vi "Funnel_ToolPath_Testing.vi"() -> ()   [LabVIEW 2020]
panel:
  out "XY Graph 2":cluster{cluster{dbl, dbl}[]}[](graph)
  out "Array":cluster{dbl, dbl}[](array[cluster])
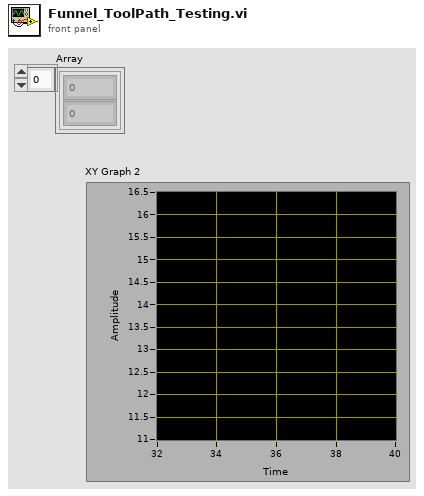
[diagram p1: front panel]
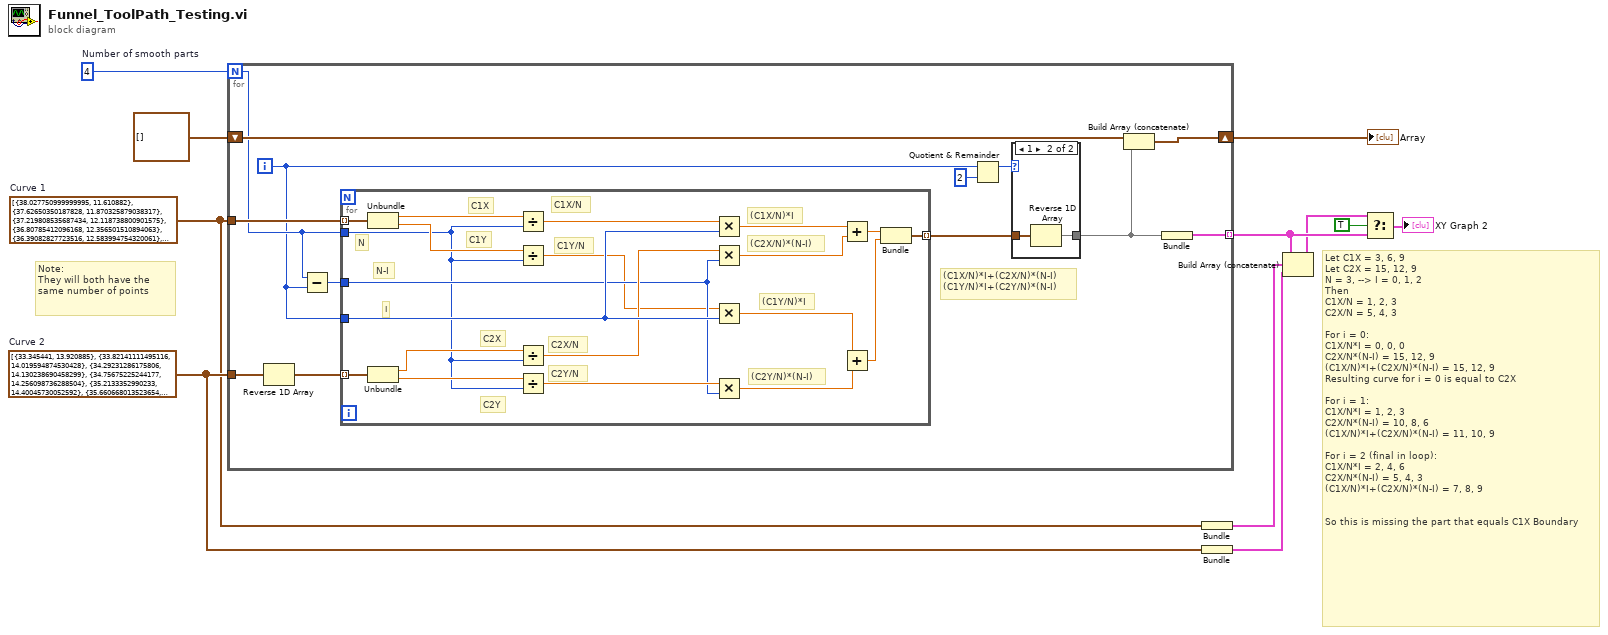
[diagram p0: block diagram]
diagram:
  w10 = 4  # Number of smooth parts
  w5 = cluster{"X":dbl, "Y":dbl}[] [{"X"=38.027750999999995, "Y"=11.610882}, {"X"=37.62650350187828, "Y"=11.870325879038317}, {"X"=37.219808535687434, "Y"=12.118738800901575}, {"X"=36.80785412096168, "Y"=12.356501510894063}, {"X"=36.39082827723516, "Y"=12.583994754320061}, {"X"=35.968919024042066, "Y"=12.801599276483847}, {"X"=35.5423143809166, "Y"=13.009695822689707}, {"X"=35.111202367392934, "Y"=13.208665138241921}, {"X"=34.67577100300526, "Y"=13.398887968444779}, {"X"=34.236208307287754, "Y"=13.580745058602556}, {"X"=33.792702299774604, "Y"=13.754617154019535}, {"X"=33.345441, "Y"=13.920885}]  # Curve 1
  w8 = cluster{"X":dbl, "Y":dbl}[] [{"X"=33.345441, "Y"=13.920885}, {"X"=33.82141111495116, "Y"=14.019594874530428}, {"X"=34.29231286175806, "Y"=14.130238690458299}, {"X"=34.75675225244177, "Y"=14.256098736288504}, {"X"=35.2133352990233, "Y"=14.40045730052592}, {"X"=35.660668013523654, "Y"=14.566596671675429}, {"X"=36.09735640796393, "Y"=14.757799138241921}, {"X"=36.52200649436513, "Y"=14.977346988730275}, {"X"=36.933224284748306, "Y"=15.22852251164538}, {"X"=37.329615791134486, "Y"=15.51460799549211}, {"X"=37.7097870255447, "Y"=15.838885728775356}, {"X"=38.072343999999994, "Y"=16.204638}]  # Curve 2
  # "Let C1X = 3, 6, 9\nLet C2X = 15, 12, 9\nN = 3, --> I = 0, 1, 2\nThen \nC1X/N = 1, 2, 3\nC2X/N = 5, 4, 3\n\nFor i = 0:\nC1X/N*I = 0, 0, 0\nC2X/N*(N-I) = 15, 12, 9\n(C1X/N)*I+(C2X/N)*(N-I) = 15, 12, 9\nResulting curve for i = 0 is equal to C2X\n\nFor i = 1:\nC1X/N*I = 1, 2, 3\nC2X/N*(N-I) = 10, 8, 6\n(C1X/N)*I+(C2X/N)*(N-I) = 11, 10, 9\n\nFor i = 2 (final in loop):\nC1X/N*I = 2, 4, 6\nC2X/N*(N-I) = 5, 4, 3\n(C1X/N)*I+(C2X/N)*(N-I) = 7, 8, 9\n\n\nSo this is missing the part that equals C1X Boundary"
  # "Note:\nThey will both have the same number of points"
  n1 = for {
    N: w10 -> [w17]
    tunnel: w8 -> [w19]
    shift-right: [w13] -> w9
    shift-left: cluster{dbl, dbl}[] [] -> [w23]
    tunnel: w5 -> [w18]
    tunnel: [w14] -> w3 mode=indexing
    i -> [w16]
    # "(C1X/N)*I+(C2X/N)*(N-I)\n(C1Y/N)*I+(C2Y/N)*(N-I)"
    n2 = Reverse 1D Array(array=w19) -> (reversed array=w22:cluster{"X":dbl, "Y":dbl}[])
    n3 = Subtract(x=w17, y=w16) -> (x-y=w24:i32)
    n4 = for {
      tunnel: w18 -> [w47] mode=indexing
      tunnel: w22 -> [w46] mode=indexing
      tunnel: w16 -> [w42]
      tunnel: w24 -> [w37]
      tunnel: [w32] -> w15 mode=indexing
      tunnel: w17 -> [w31]
      # "C2Y"
      # "I"
      # "N"
      # "N-I"
      # "(C2Y/N)*(N-I)"
      # "C2Y/N"
      # "(C2X/N)*(N-I)"
      # "C2X/N"
      # "C2X"
      # "(C1Y/N)*I"
      # "C1Y/N"
      # "C1Y"
      # "(C1X/N)*I"
      # "C1X/N"
      # "C1X"
      n5 = Unbundle(w47) -> ("X"=w45:dbl, "Y"=w43:dbl)
      n6 = Unbundle(w46) -> ("X"=w41:dbl, "Y"=w40:dbl)
      n7 = Divide(x=w45, y=w31) -> (x/y=w44:dbl)
      n8 = Divide(x=w43, y=w31) -> (x/y=w29:dbl)
      n9 = Divide(x=w41, y=w31) -> (x/y=w39:dbl)
      n10 = Divide(x=w40, y=w31) -> (x/y=w38:dbl)
      n11 = Multiply(x=w44, y=w42) -> (x*y=w36:dbl)
      n12 = Multiply(x=w39, y=w37) -> (x*y=w35:dbl)
      n13 = Multiply(x=w29, y=w42) -> (x*y=w34:dbl)
      n14 = Multiply(x=w38, y=w37) -> (x*y=w28:dbl)
      n15 = Add(x=w36, y=w35) -> (x+y=w33:dbl)
      n16 = Add(x=w34, y=w28) -> (x+y=w30:dbl)
      n17 = Bundle(w33, w30) -> (w32:cluster{dbl, dbl})  [unwired: 1 in]
    }
    n18 = Quotient & Remainder(x=w16, y=2) -> (x-y*floor(x/y)=w20:i32)  [unwired: 1 out]
    n19 = case shown="1" w20 {
      tunnel: w15 -> [w25 w27]
      tunnel: [w25 w26] -> w12
      frame 0, Default {
      }
      frame 1 {
        n20 = Reverse 1D Array(array=w27) -> (reversed array=w26:cluster{dbl, dbl}[])
      }
    }
    n21 = Build Array (concatenate)(w23, w12) -> (w13:cluster{dbl, dbl}[])
    n22 = Bundle(w12) -> (w14:cluster{cluster{dbl, dbl}[]})  [unwired: 1 in]
  }
  "Array" <- w9
  n23 = Bundle("Curve 1"=w5) -> (w4:cluster{"Curve 1":cluster{"X":dbl, "Y":dbl}[]})  [unwired: 1 in]
  n24 = Bundle("Curve 2"=w8) -> (w1:cluster{"Curve 2":cluster{"X":dbl, "Y":dbl}[]})  [unwired: 1 in]
  n25 = Build Array (concatenate)(w3, w4, w1) -> (w2:cluster{"Curve 2":cluster{"X":dbl, "Y":dbl}[]}[])
  n26 = Select(t=w2, s=TRUE, f=w3) -> (s? t:f=→"XY Graph 2":cluster{"Curve 2":cluster{"X":dbl, "Y":dbl}[]}[])
